vi "user32_GetDesktopWindow.vi"(11 "错误输入（无错误）":errorcluster) -> (4 "hWnd":u32, 6 "success?":bool, 15 "错误输出":errorcluster)   [LabVIEW 2011]
doc: "该函数返回桌面窗口的句柄。桌面窗口覆盖整个屏幕。桌面窗口是一个要在其上绘制所有的图标和其他窗口的区域。"
uses:
  user32.dll
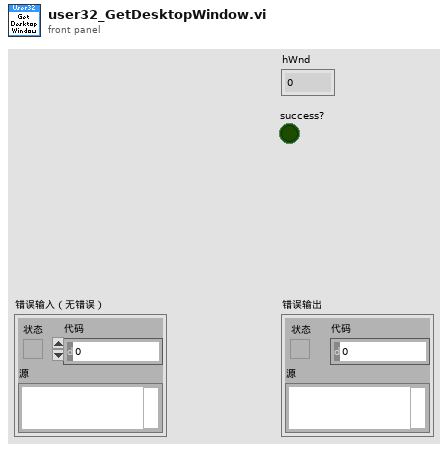
[diagram p1: front panel]
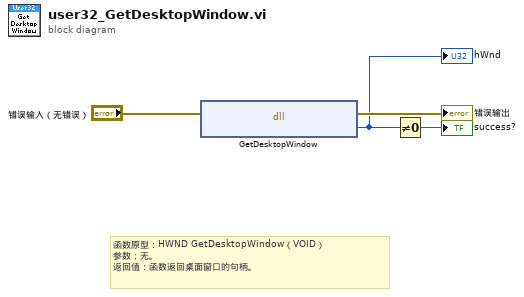
[diagram p0: block diagram]
diagram:
  # "函数原型：HWND GetDesktopWindow（VOID）\n参数：无。\n返回值：函数返回桌面窗口的句柄。"
  n1 = dll-call lib="user32.dll" fn="GetDesktopWindow"(error in="错误输入（无错误）") -> (error out=→"错误输出":errorcluster, "hWnd"=w1:u32)  [unwired: 2 in, 1 out]
  "hWnd" <- w1
  n2 = Not Equal To 0?(x=w1) -> (x != 0?=→"success?":bool)
